vi "audio.vi"() -> ()   [LabVIEW 2010]
uses:
  <vilib>/measure/NI_MABase.lvlib
panel:
  in  "Sound":bool
  in  "stop":bool
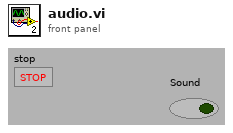
[diagram p1: front panel]
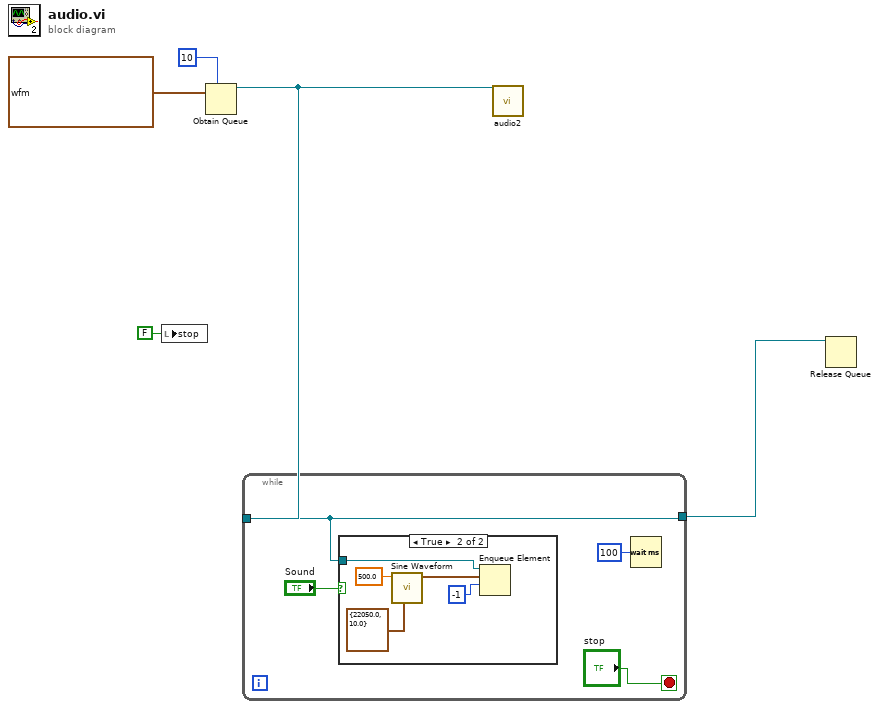
[diagram p0: block diagram]
diagram:
  n1 = local write "stop"(FALSE ("stop")) -> ()
  n2 = Obtain Queue(max queue size (-1, unlimited)=10, element data type=waveform(dbl) {"t0"=timestamp(0 s since 1904-01-01), "dt"=1.0, "Y"=[]} ("Waveform")) -> (queue out=w1:refnum<queue>)  [unwired: 3 in, 2 out]
  n3 = while {
    tunnel: w1 -> [w6]
    tunnel: [w6] -> w4
    stop <- "stop" stop-if-true
    n4 = case shown="True" "Sound" {
      tunnel: w6 -> [_ w14]
      frame False {
      }
      frame True {
        n5 = call <vilib>:"Sine Waveform.vi"("sampling info"=cluster{"Fs":dbl, "#s":dbl} {"Fs"=22050.0, "#s"=10.0}, "frequency"=500.0) -> ("signal out"=w13:waveform(dbl))  [unwired: 8 in, 1 out]
        n6 = Enqueue Element(queue=w14, element=w13, timeout in ms (-1)=-1) -> ()  [unwired: 1 in, 3 out]
      }
    }
    n7 = Wait (ms)(milliseconds to wait=u32 100) -> ()  [unwired: 1 out]
  }
  n8 = call "audio2.vi"("queue out"=w1) -> ()  [unwired: 11 in]
  n9 = Release Queue(queue=w4) -> ()  [unwired: 2 in, 3 out]
